vi "Main.vi"() -> ()   [LabVIEW 2017]
uses:
  Engine/Engine.lvclass
panel:
  in  "Save to VIs":bool
  in  "VIs":string[][](table)
  in  "Library Path":path
  in  "Load Library":bool
  in  "Export to CSV":bool
  in  "Import from CSV":bool
  in  "Exit":bool
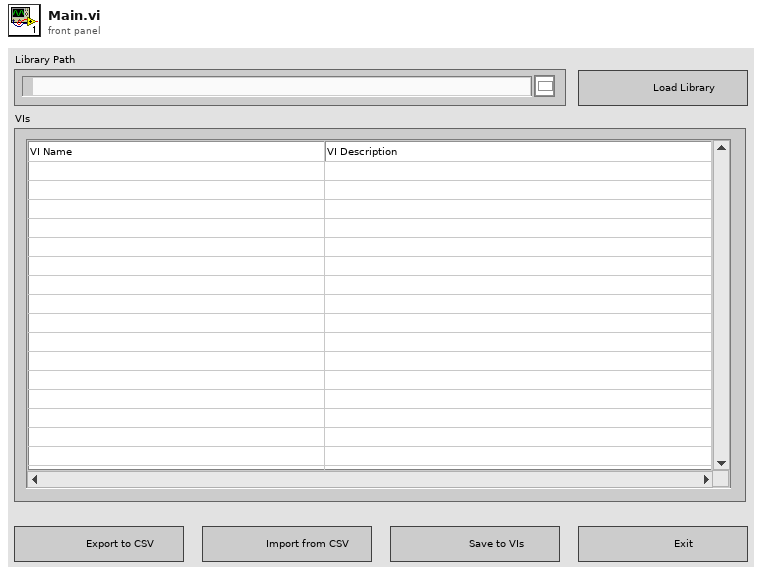
[diagram p1: front panel]
types:
  T1 = typedef "Engine.lvclass/VI Information.ctl" = cluster{"VI Name":string, "VI Description":string}
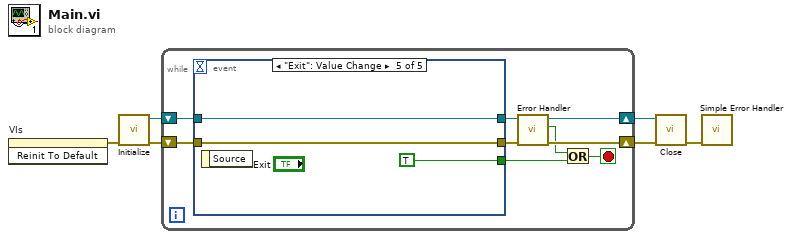
[diagram p0: block diagram]
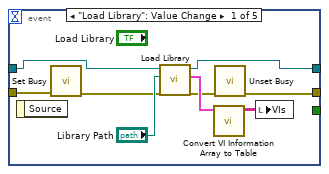
[diagram p2: hidden frame]
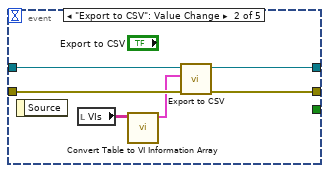
[diagram p3: hidden frame]
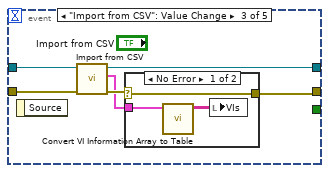
[diagram p4: hidden frame]
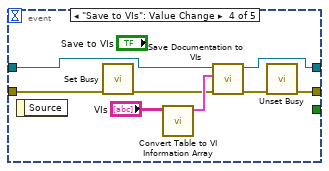
[diagram p6: hidden frame]
diagram:
  n1 = invoke on="VIs" class="Tbl (strict)" method="Reinit To Default"() -> (error out=w6:errorcluster)  [unwired: 3 in, 2 out]
  n2 = call "Initialize.vi"("error in"=w6) -> ("error out"=w5:errorcluster, "Engine out"=w4:refnum<class "Engine.lvclass">)  [unwired: 9 in]
  n3 = while {
    shift-right: [w10] -> w3
    shift-left: w5 -> [w13]
    shift-right: [w8] -> w1
    shift-left: w4 -> [w11]
    stop <- w15 stop-if-true
    n4 = event shown="[4] \"Exit\": Value Change" {
      selector: _ -> [_ _ _ _ _]
      dyn-events: _ -> [_ _ _ _ _]
      timeout: _ -> [_ _ _ _ _]
      tunnel: [w16 w29 w32 w41 w50] -> w14
      tunnel: w13 -> [w19 w30 w36 w48 w50]
      tunnel: [_ _ _ _ TRUE] -> w12
      tunnel: [w23 w27 w34 w45 w49] -> w9
      tunnel: w11 -> [w22 w28 w35 w46 w49]
      event "Load Library": Value Change {
        n5 = event-data() -> ()  [unwired: 1 in, 1 out]
        n6 = call <vilib>:"Set Busy.vi"("error in (no error)"=w19) -> ("error out"=w18:errorcluster)  [unwired: 9 in, 1 out]
        n7 = call "Load Library.vi"("error in"=w18, "Library Path"="Library Path", "Engine in"=w22) -> ("error out"=w17:errorcluster, "VIs and Descriptions Array"=w21:T1[], "Engine out"=w23:refnum<class "Engine.lvclass">)  [unwired: 6 in]
        n8 = call "Convert VI Information Array to Table.vi"("VI Information Array"=w21) -> ("Array Out"=w20:string[][])  [unwired: 10 in]
        n9 = call <vilib>:"Unset Busy.vi"("error in (no error)"=w17) -> ("error out"=w16:errorcluster)  [unwired: 10 in]
        n10 = local write "VIs"(w20) -> ()
      }
      event "Export to CSV": Value Change {
        n11 = event-data() -> ()  [unwired: 1 in, 1 out]
        n12 = local read "VIs"() -> (w26:string[][])
        n13 = call "Convert Table to VI Information Array.vi"("Array Out"=w26) -> ("VI Information Array"=w25:T1[])  [unwired: 10 in]
        n14 = call "Export to CSV.vi"("error in"=w30, "VI Information Array"=w25, "Engine in"=w28) -> ("error out"=w29:errorcluster, "Engine out"=w27:refnum<class "Engine.lvclass">)  [unwired: 7 in]
      }
      event "Import from CSV": Value Change {
        n15 = event-data() -> ()  [unwired: 1 in, 1 out]
        n16 = call "Import from CSV.vi"("error in"=w36, "Engine in"=w35) -> ("error out"=w33:errorcluster, "VI Information Array"=w31:T1[], "Engine out"=w34:refnum<class "Engine.lvclass">)  [unwired: 7 in]
        n17 = case shown="No Error" w33 {
          selector: w33 -> [w38 w40]
          tunnel: [w38 w40] -> w32
          tunnel: w31 -> [w39 _]
          frame No Error {
            n18 = call "Convert VI Information Array to Table.vi"("VI Information Array"=w39) -> ("Array Out"=w37:string[][])  [unwired: 10 in]
            n19 = local write "VIs"(w37) -> ()
          }
          frame Error {
          }
        }
      }
      event "Save to VIs": Value Change {
        n20 = event-data() -> ()  [unwired: 1 in, 1 out]
        n21 = call <vilib>:"Set Busy.vi"("error in (no error)"=w48) -> ("error out"=w42:errorcluster)  [unwired: 9 in, 1 out]
        n22 = call "Convert Table to VI Information Array.vi"("Array Out"="VIs") -> ("VI Information Array"=w43:T1[])  [unwired: 10 in]
        n23 = call "Save Documentation to VIs.vi"("error in"=w42, "VI Information Array"=w43, "Engine in"=w46) -> ("error out"=w47:errorcluster, "Engine out"=w45:refnum<class "Engine.lvclass">)  [unwired: 7 in]
        n24 = call <vilib>:"Unset Busy.vi"("error in (no error)"=w47) -> ("error out"=w41:errorcluster)  [unwired: 10 in]
      }
      event "Exit": Value Change {
        n25 = event-data() -> ()  [unwired: 1 in, 1 out]
      }
    }
    n26 = call "Error Handler.vi"("error in"=w14, "Engine in"=w9) -> ("error out"=w10:errorcluster, "Stop Application"=w7:bool, "Engine out"=w8:refnum<class "Engine.lvclass">)  [unwired: 7 in]
    n27 = Or(x=w7, y=w12) -> (x .or. y?=w15:bool)
  }
  n28 = call "Close.vi"("error in"=w3, "Engine in"=w1) -> ("error out"=w2:errorcluster)  [unwired: 9 in]
  n29 = call <vilib>:"Simple Error Handler.vi"("error in (no error)"=w2) -> ()  [unwired: 4 in, 5 out]
